vi "DataLogger.vi"() -> ()   [LabVIEW 2021]
panel:
  out "App:Default Data Directory":path
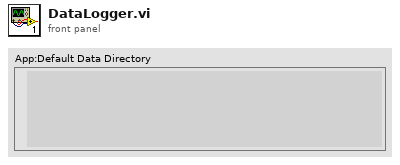
[diagram p1: front panel]
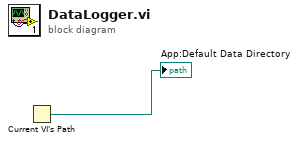
[diagram p0: block diagram]
diagram:
  n1 = Current VI's Path() -> (path=→"App:Default Data Directory":path)
